vi "Image_instruction.vi"(11 "3P4S?":bool) -> (3 "Array":string[][](array[string]))   [LabVIEW 2020]
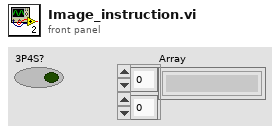
[diagram p1: front panel]
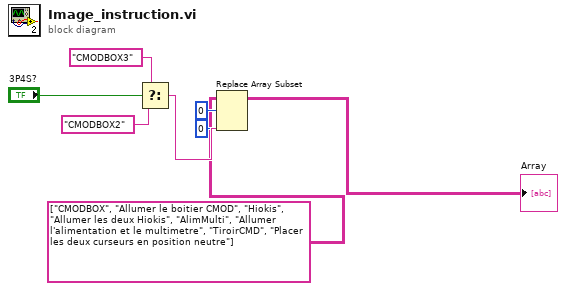
[diagram p0: block diagram]
diagram:
  n1 = Select(t="CMODBOX3", s="3P4S?", f="CMODBOX2") -> (s? t:f=w8:string)
  n2 = Replace Array Subset(array=string[][] [["CMODBOX", "Allumer le boitier CMOD"], ["Hiokis", "Allumer les deux Hiokis"], ["AlimMulti", "Allumer l'alimentation et le multimetre"], ["TiroirCMD", "Placer les deux curseurs en position neutre"]], new element=w8, index (row)=0, index (col)=0 ("disabled index (col)")) -> (→"Array":string[][])
